vi "Test Accumulate Case Execution Time.vi"(8 "error in (no error)":errorcluster, 11 "Test Result Tree Test in":refnum<class "Test Result Tree Test.lvclass">) -> (0 "error out":errorcluster, 3 "Test Result Tree Test out":refnum<class "Test Result Tree Test.lvclass">)   [LabVIEW 2020, in "Test Result Tree Test.lvclass"]
uses:
  Test Result Tree Test.lvclass
  C:/Program Files (x86)/National Instruments/LabVIEW 2020/vi.lib/Astemes/LUnit/Test Case.lvclass
  Test Result Tree/Test Result Tree V2.lvclass
  C:/Git/astemes-lunit/source/Rewrite Project/Test Tree/Test Tree.lvclass
  Result/Result.ctl
  Result/Status.ctl
  Result/Type.ctl
  <vilib>/Astemes/LUnit/Test Case.lvclass/Test Case.ctl
  b37c0ee5-4232-4b66-8e49-fde6ff6ab9c1.vi
  <vilib>/Astemes/LUnit/Palette/Pass.vi
  <vilib>/Astemes/LUnit/Palette/Fail.vi
  <vilib>/Astemes/LUnit/Compare Variants.vi
  <vilib>/Astemes/LUnit/Describe Comparison.vi
  <vilib>/Astemes/LUnit/Set Assertion Type.vi
  <vilib>/Astemes/LUnit/Add test result.vi
  <vilib>/Astemes/LUnit/Variant to string.vi
  <vilib>/Astemes/LUnit/LUnit Record Assertion Result.vi
  <vilib>/Astemes/LUnit/LUnit Aggregate Assertion Results.vi
  <vilib>/Astemes/LUnit/Method Result/LUnit Merge Status.vi
  <vilib>/Astemes/LUnit/LUnit Concatenate result strings.vi
  <vilib>/Utility/Data Type/Get Type Information.vi
  <vilib>/Utility/LVClass/Get LV Class Name.vi
  Test Result Tree Test.lvclass/Test Result Tree Test.ctl
  Test Tree/Test Tree.lvclass
  Result/Result.lvlib
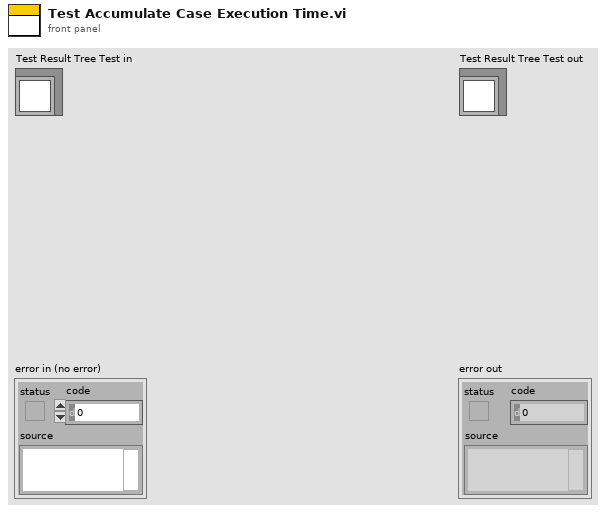
[diagram p1: front panel]
types:
  T1 = typedef "Result.lvlib/Result.ctl" = cluster{"Name":string, "Message":string, "Description":string, "Status":T2, "Result Type":T3, "Execution Time":dbl}
  T2 = typedef "Result.lvlib/Status.ctl" = enum16{"", "Passed", "Failed", "Error", "Skipped", "Setup Error", "Broken", "Teardown Error"}
  T3 = typedef "Result.lvlib/Type.ctl" = enum16{"Method", "Case", "Suite", "Pass", "Fail", "Skip", "Pass if", "Fail if", "Pass if Error", "Fail if Error", "Pass if Equal", "Fail if Equal"}
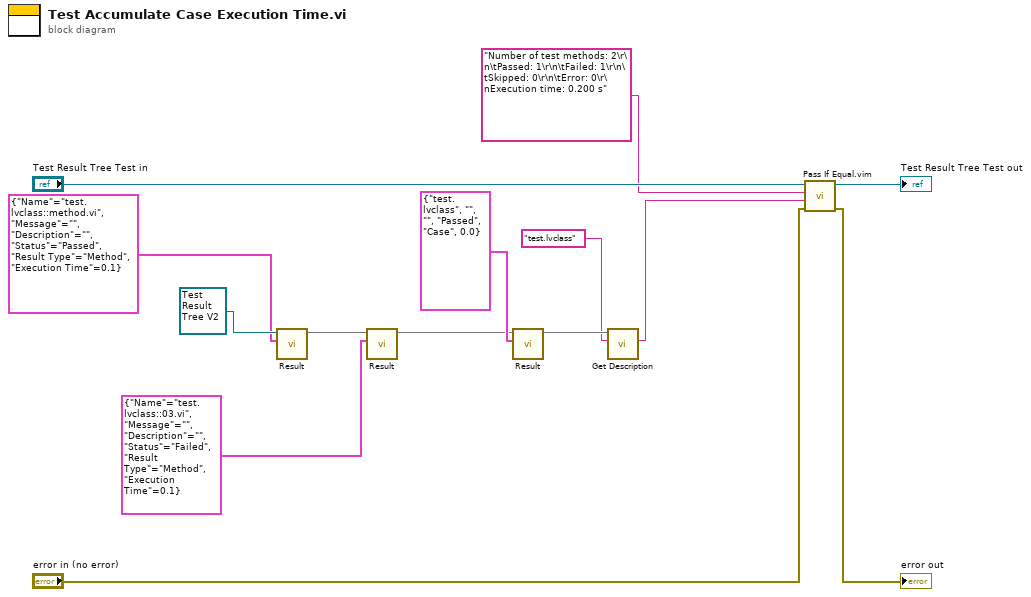
[diagram p0: block diagram]
diagram:
  n1 = call-dynamic "Result.vi"("Result"=T1 {"Name"="test.lvclass::method.vi", "Message"="", "Description"="", "Status"=enum."Passed", "Result Type"=enum."Method", "Execution Time"=0.1}, "Test Result Tree V2 in"=refnum<class "Test Result Tree V2.lvclass"> refnum ("Test Result Tree V2.lvclass")) -> (3:w3)  [unwired: 8 in, 1 out]
  n2 = call-dynamic "Result.vi"("Result"=T1 {"Name"="test.lvclass::03.vi", "Message"="", "Description"="", "Status"=enum."Failed", "Result Type"=enum."Method", "Execution Time"=0.1}, "Test Result Tree V2 in"=w3) -> (3:w2)  [unwired: 8 in, 1 out]
  n3 = call-dynamic "Result.vi"("Result"=T1 {"Name"="test.lvclass", "Message"="", "Description"="", "Status"=enum."Passed", "Result Type"=enum."Case", "Execution Time"=0.0}, "Test Result Tree V2 in"=w2) -> (3:w9)  [unwired: 8 in, 1 out]
  n4 = call "Get Description.vi"("Tag"="test.lvclass" ("Case"), "Test Tree In"=w9) -> ("Description"=w7:string)  [unwired: 6 in, 3 out]
  n5 = call "Pass If Equal.vim"("error in (no error)"="error in (no error)", "Actual"=w7, "Expected"="Number of test methods: 2\r\n\tPassed: 1\r\n\tFailed: 1\r\n\tSkipped: 0\r\n\tError: 0\r\nExecution time: 0.200 s" ("format string"), "LUnit Test Case In"="Test Result Tree Test in") -> ("error out"=→"error out":errorcluster, "LUnit Test Case Out"=→"Test Result Tree Test out":refnum<class "Test Result Tree Test.lvclass">)  [unwired: 6 in]
